vi "ALONE_RAMPAVOLT.vi"(6 "Refresco(s)":dbl=0.1 caption="Elapsed Time (s)" format="%.1f", 8 "error in (no error)":errorcluster) -> (0 "Error Out":errorcluster, 7 "Enable":bool=TRUE)   [LabVIEW 2017]
uses:
  <vilib>/Analysis/baseanly.llb/Mean (DBL).vi
  cRIO_ZNB_AMI_GLOBALES.vi
  <vilib>/gmath/NI_Gmath.lvlib
  <vilib>/Analysis/NI_AALBase.lvlib
panel:
  in  "Send":bool
  in  "q":i32=10 caption="Puntos, q" format="%#.0f"
  out "Array":dbl[](array[numeric])
  out "V Stable (T:yes)":bool caption="Stable"
  out "Voltage Status":i32(ring) items=["VoltageUnknown", "Stable", "Tracking"]
  out "Num 1":i32
  out "Num 2":i32
  out "SetPoint(V).":dbl format="%.2f"
  in  "Setpoint(V)":dbl format="%.2f"
  in  "Rate(V/min)":dbl=0.1 format="%.2f"
  out "Voltage(V).":dbl format="%.2f"
  out "ERROR":bool
  out "Date":string caption="asd"
  out "Time":string
  in  "Refresh":bool
  in  "stop":bool
  # "Rampa de voltaje (Aout1)"
  # "STATUS"
  # "SETTINGS"
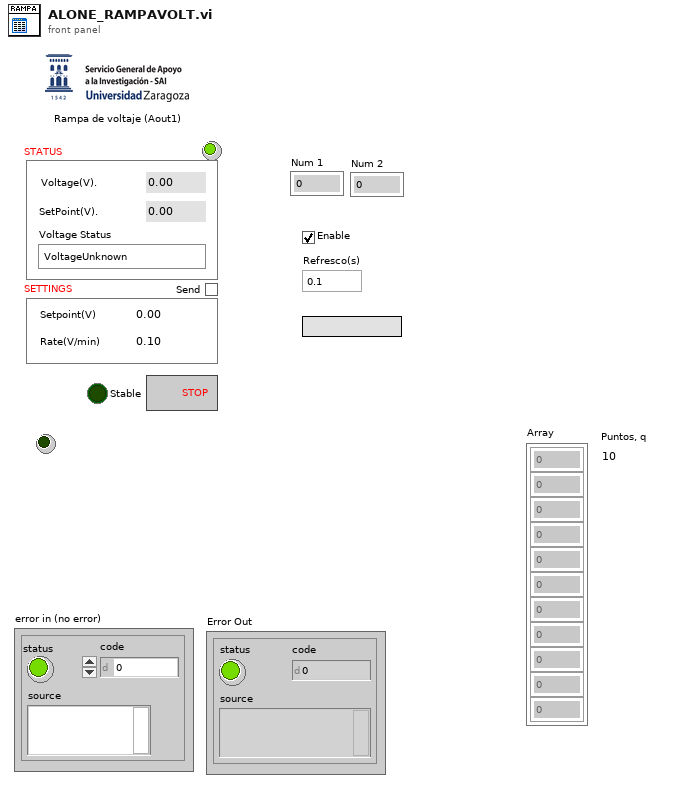
[diagram p1: front panel]
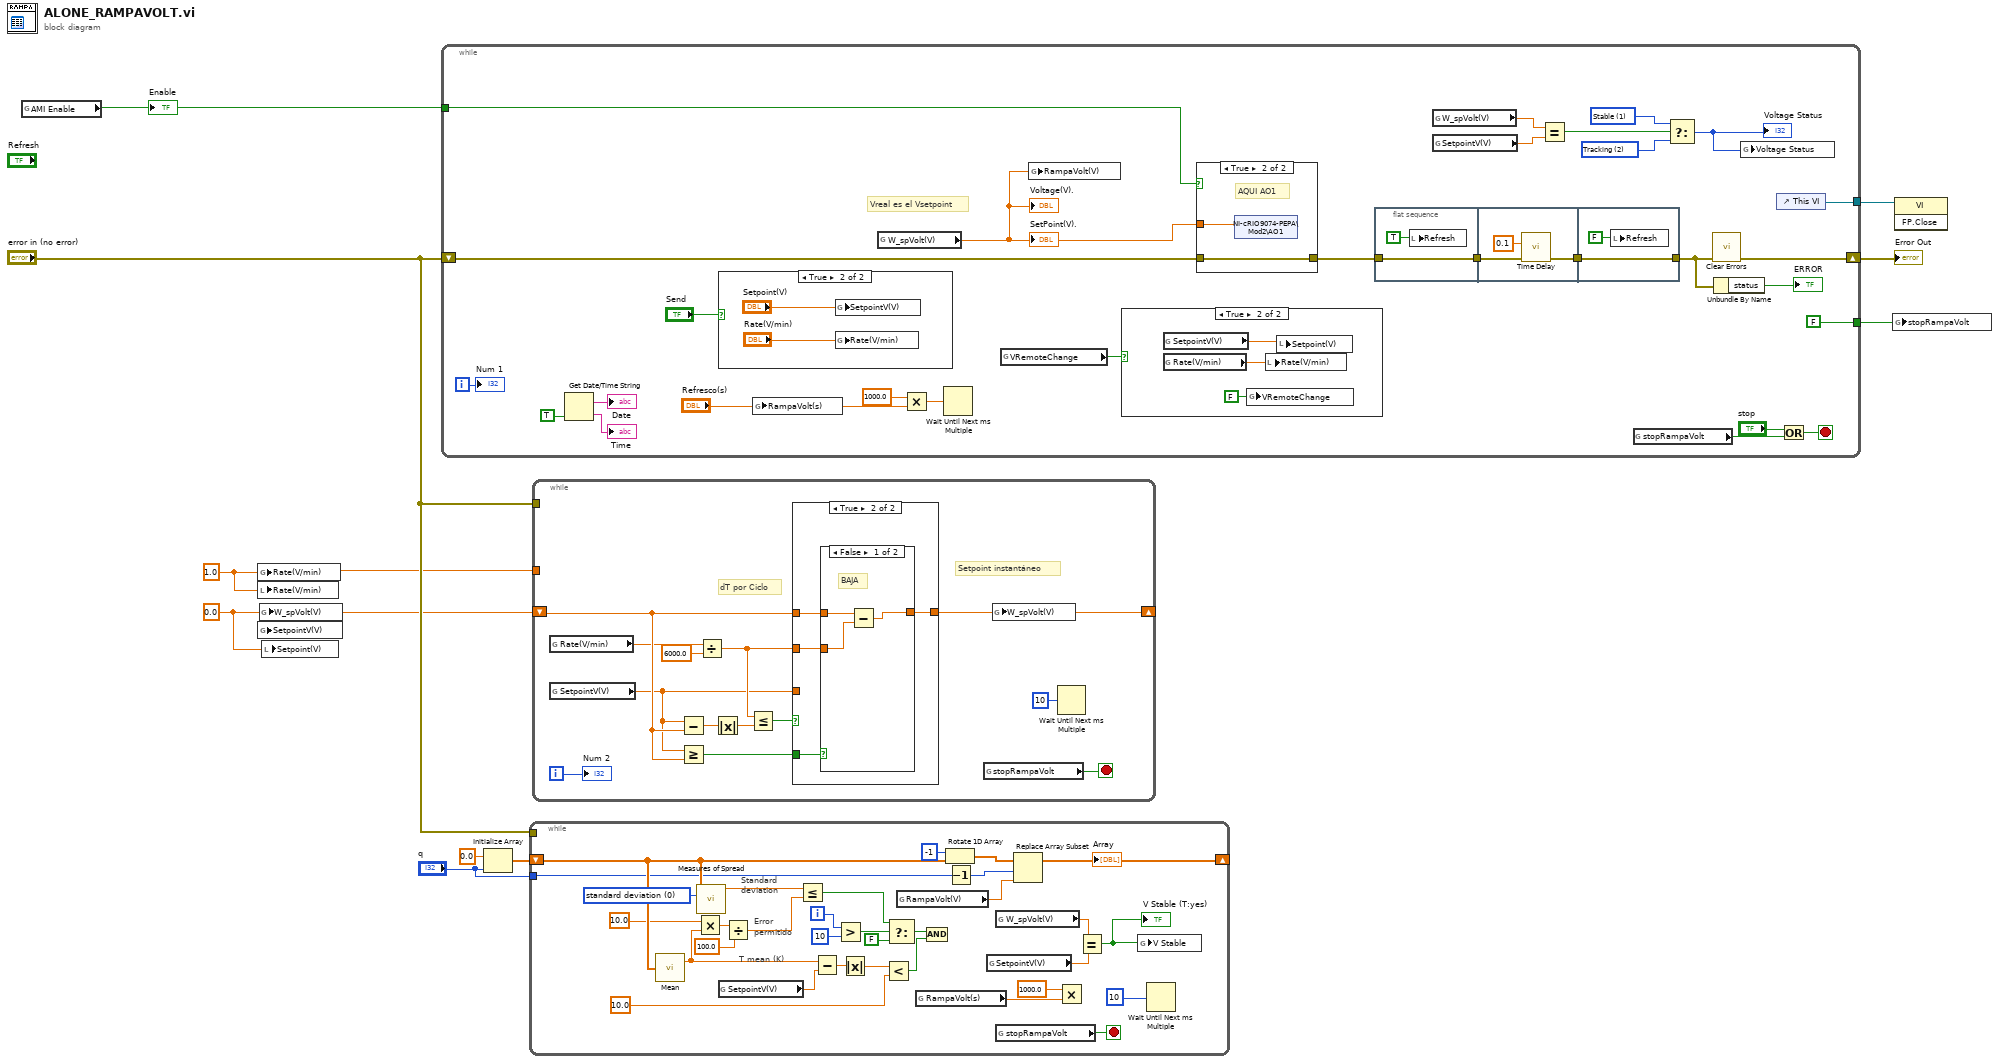
[diagram p0: block diagram]
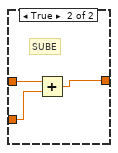
[diagram p3: hidden frame]
diagram:
  w1 = 0.0 ("W_spTemp(K)")
  w2 = 1.0 ("Rate(K/min)")
  n1 = global read "cRIO_ZNB_AMI_GLOBALES.vi" "AMI Enable"() -> (w7:bool)
  "Enable" <- w7
  n2 = global write "cRIO_ZNB_AMI_GLOBALES.vi" "Rate(V/min)"(w2) -> ()
  n3 = local write "Rate(V/min)"(w2) -> ()
  n4 = global write "cRIO_ZNB_AMI_GLOBALES.vi" "SetpointV(V)"(w1) -> ()
  n5 = global write "cRIO_ZNB_AMI_GLOBALES.vi" "W_spVolt(V)"(w1) -> ()
  n6 = local write "Setpoint(V)"(w1) -> ()
  n7 = while {
    shift-right: [w28] -> w8
    shift-left: "error in (no error)" -> [w14]
    tunnel: [FALSE ("stop")] -> w9
    tunnel: [w33] -> w10
    tunnel: w7 -> [w23]
    i -> [w24]
    stop <- w37 stop-if-true
    w12 = 2 items=["VoltageUnknown", "Stable", "Tracking"] ("Voltage Status")
    w11 = 1 items=["VoltageUnknown", "Stable", "Tracking"] ("Voltage Status")
    # "Vreal es el Vsetpoint"
    n8 = Get Date/Time String(want seconds? (F)=TRUE) -> (date string=→"Date":string, time string=→"Time":string)  [unwired: 2 in]
    n9 = case shown="True" "Send" {
      frame False {
      }
      frame True {
        n10 = global write "cRIO_ZNB_AMI_GLOBALES.vi" "SetpointV(V)"("Setpoint(V)") -> ()
        n11 = global write "cRIO_ZNB_AMI_GLOBALES.vi" "Rate(V/min)"("Rate(V/min)") -> ()
      }
    }
    n12 = global write "cRIO_ZNB_AMI_GLOBALES.vi" "RampaVolt(s)"("Refresco(s)") -> ()
    n13 = global read "cRIO_ZNB_AMI_GLOBALES.vi" "W_spVolt(V)"() -> (w13:dbl)
    "Voltage(V)." <- w13
    "SetPoint(V)." <- w13
    n14 = Multiply(x=1000.0, y="Refresco(s)") -> (x*y=w29:dbl)
    n15 = Wait Until Next ms Multiple(millisecond multiple=w29) -> ()  [unwired: 1 out]
    n16 = global read "cRIO_ZNB_AMI_GLOBALES.vi" "VRemoteChange"() -> (w15:bool)
    n17 = global write "cRIO_ZNB_AMI_GLOBALES.vi" "RampaVolt(V)"(w13) -> ()
    n18 = case shown="True" w15 {
      frame False {
      }
      frame True {
        n19 = global read "cRIO_ZNB_AMI_GLOBALES.vi" "SetpointV(V)"() -> (w42:dbl)
        n20 = global read "cRIO_ZNB_AMI_GLOBALES.vi" "Rate(V/min)"() -> (w41:dbl)
        n21 = global write "cRIO_ZNB_AMI_GLOBALES.vi" "VRemoteChange"(FALSE ("TRemoteChange")) -> ()
        n22 = local write "Rate(V/min)"(w41) -> ()
        n23 = local write "Setpoint(V)"(w42) -> ()
      }
    }
    n24 = case shown="True" w23 {
      tunnel: w13 -> [_ w46]
      tunnel: w14 -> [w45 w47]
      tunnel: [w45 w47] -> w22
      frame False {
      }
      frame True {
        # "AQUI AO1"
        n25 = shared-variable "NI-cRIO9074-PEPA\\Mod2\\AO1"(w46) -> ()  [unwired: 1 in, 1 out]
      }
    }
    n26 = flat-sequence {
      tunnel: w22 -> [w48]
      tunnel: [w48] -> w27
      tunnel: w27 -> [w51]
      tunnel: [w50] -> w26
      tunnel: [w53] -> w25
      tunnel: w26 -> [w53]
      frame #0 {
        n27 = local write "Refresh"(TRUE ("Refresh")) -> ()
      }
      frame #1 {
        n28 = call "Time Delay"("error in (no error)"=w51, "Delay Time (s)"=0.1) -> ("error out"=w50:errorcluster)  [unwired: 9 in]
      }
      frame #2 {
        n29 = local write "Refresh"(FALSE ("Refresh")) -> ()
      }
    }
    n30 = global read "cRIO_ZNB_AMI_GLOBALES.vi" "W_spVolt(V)"() -> (w19:dbl)
    n31 = global read "cRIO_ZNB_AMI_GLOBALES.vi" "SetpointV(V)"() -> (w18:dbl)
    n32 = Equal?(x=w19, y=w18) -> (x = y?=w17:bool)
    n33 = global read "cRIO_ZNB_AMI_GLOBALES.vi" "stopRampaVolt"() -> (w32:bool)
    n34 = Select(t=w11, s=w17, f=w12) -> (s? t:f=w20:i32)
    "Voltage Status" <- w20
    n35 = call <vilib>:"Clear Errors.vi"("error in (no error)"=w25) -> ("error out"=w28:errorcluster)  [unwired: 5 in, 1 out]
    n36 = Unbundle By Name(w25) -> ("status"=→"ERROR":bool)
    n37 = global write "cRIO_ZNB_AMI_GLOBALES.vi" "Voltage Status"(w20) -> ()
    n38 = control-ref of="This VI"() -> (w33:refnum<vi>)
    n39 = Or(x="stop", y=w32) -> (x .or. y?=w37:bool)
    "Num 1" <- w24
  }
  "Error Out" <- w8
  n40 = Initialize Array(0.0 ("element"), "q") -> (w6:dbl[])
  n41 = while {
    tunnel: "q" -> [w67]
    shift-right: [w82] -> _
    shift-left: w6 -> [w68]
    tunnel: "error in (no error)" -> [_]
    i -> [w61]
    stop <- w86 stop-if-true
    w72 = 0 items=["standard deviation", "range", "mean absolute deviation", "interquartile range"] ("type")
    # "Error\npermitido"
    # "Standard\ndeviation"
    # "T mean (K)"
    n42 = call-poly <vilib>:"Mean.vi"("X"=w68) -> ("mean"=w66:dbl)  [unwired: 1 out]
    n43 = Multiply(x=10.0, y=w66) -> (x*y=w77:dbl)
    n44 = call <vilib>:"Measures of Spread.vi"("type"=w72, "x array"=w68) -> ("spread value"=w81:dbl)  [unwired: 8 in, 1 out]
    n45 = global read "cRIO_ZNB_AMI_GLOBALES.vi" "SetpointV(V)"() -> (w65:dbl)
    n46 = Divide(x=w77, y=100.0) -> (x/y=w76:dbl)
    n47 = Less Or Equal?(x=w81, y=w76) -> (x <= y?=w79:bool)
    n48 = Subtract(x=w66, y=w65) -> (x-y=w75:dbl)
    n49 = Greater?(x=w61, y=10) -> (0:w80:bool)
    n50 = Absolute Value(x=w75) -> (abs(x)=w74:dbl)
    n51 = Less?(x=w74, y=10.0 ("x")) -> (x < y?=w73:bool)
    n52 = Select(t=w79, s=w80, f=FALSE ("TdownStable (T:yes)")) -> (s? t:f=w78:bool)
    n53 = global read "cRIO_ZNB_AMI_GLOBALES.vi" "RampaVolt(V)"() -> (w64:dbl)
    n54 = global read "cRIO_ZNB_AMI_GLOBALES.vi" "RampaVolt(s)"() -> (w63:dbl)
    n55 = And(x=w78, y=w73) -> ()  [unwired: 1 out]
    n56 = Rotate 1D Array(1:w68, 2:-1 ("n")) -> (0:w84:dbl[])
    n57 = Decrement(x=w67) -> (x-1=w85:i32)
    n58 = global read "cRIO_ZNB_AMI_GLOBALES.vi" "SetpointV(V)"() -> (w56:dbl)
    n59 = global read "cRIO_ZNB_AMI_GLOBALES.vi" "W_spVolt(V)"() -> (w57:dbl)
    n60 = global read "cRIO_ZNB_AMI_GLOBALES.vi" "stopRampaVolt"() -> (w86:bool)
    n61 = Replace Array Subset(array=w84, new element=w64, index=w85) -> (w82:dbl[])
    "Array" <- w82
    n62 = Multiply(x=1000.0, y=w63) -> ()  [unwired: 1 out]
    n63 = Equal?(x=w57, y=w56) -> (x = y?=w58:bool)
    "V Stable (T:yes)" <- w58
    n64 = global write "cRIO_ZNB_AMI_GLOBALES.vi" "V Stable"(w58) -> ()
    n65 = Wait Until Next ms Multiple(millisecond multiple=i64 10 ("Period")) -> ()  [unwired: 1 out]
  }
  n66 = while {
    shift-right: [w92] -> _
    shift-left: w1 -> [w97]
    tunnel: "error in (no error)" -> [_]
    tunnel: w2 -> [_]
    i -> [w88]
    stop <- w89 stop-if-true
    # "Setpoint instantáneo"
    # "dT por Ciclo"
    n67 = global read "cRIO_ZNB_AMI_GLOBALES.vi" "Rate(V/min)"() -> (w91:dbl)
    n68 = global read "cRIO_ZNB_AMI_GLOBALES.vi" "SetpointV(V)"() -> (w90:dbl)
    n69 = Subtract(x=w90, y=w97) -> (x-y=w96:dbl)
    n70 = Greater Or Equal?(x=w90, y=w97) -> (x >= y?=w99:bool)
    n71 = Divide(x=w91, y=6000.0) -> (x/y=w95:dbl)
    n72 = Absolute Value(x=w96) -> (abs(x)=w94:dbl)
    n73 = Less Or Equal?(x=w95, y=w94) -> (x <= y?=w93:bool)
    n74 = case shown="True" w93 {
      tunnel: w90 -> [w100 _]
      tunnel: w95 -> [_ w101]
      tunnel: w97 -> [_ w104]
      tunnel: [w100 w103] -> w92
      tunnel: w99 -> [_ w102]
      frame False {
      }
      frame True {
        n75 = case shown="False" w102 {
          tunnel: w104 -> [w106 w109]
          tunnel: [w107 w110] -> w103
          tunnel: w101 -> [w105 w108]
          frame False {
            # "BAJA"
            n76 = Subtract(x=w106, y=w105) -> (x-y=w107:dbl)
          }
          frame True {
            # "SUBE"
            n77 = Add(x=w109, y=w108) -> (x+y=w110:dbl)
          }
        }
      }
    }
    n78 = global read "cRIO_ZNB_AMI_GLOBALES.vi" "stopRampaVolt"() -> (w89:bool)
    n79 = global write "cRIO_ZNB_AMI_GLOBALES.vi" "W_spVolt(V)"(w92) -> ()
    n80 = Wait Until Next ms Multiple(millisecond multiple=i64 10 ("Period")) -> ()  [unwired: 1 out]
    "Num 2" <- w88
  }
  n81 = global write "cRIO_ZNB_AMI_GLOBALES.vi" "stopRampaVolt"(w9) -> ()
  n82 = invoke class="VI" method="FP.Close"(reference=w10) -> ()  [unwired: 2 in, 3 out]
